vi "globalSetUp.vi"(8 "error in (no error)":errorcluster, 11 "Instrument Addon Host API Tests in":refnum<class "Instrument Addon Host API Tests.lvclass">) -> (0 "error out":errorcluster, 3 "Instrument Addon Host API Tests out":refnum<class "Instrument Addon Host API Tests.lvclass">)   [LabVIEW 2019, in "Instrument Addon Host API Tests.lvclass"]
uses:
  Instrument Addon Host API Tests.lvclass
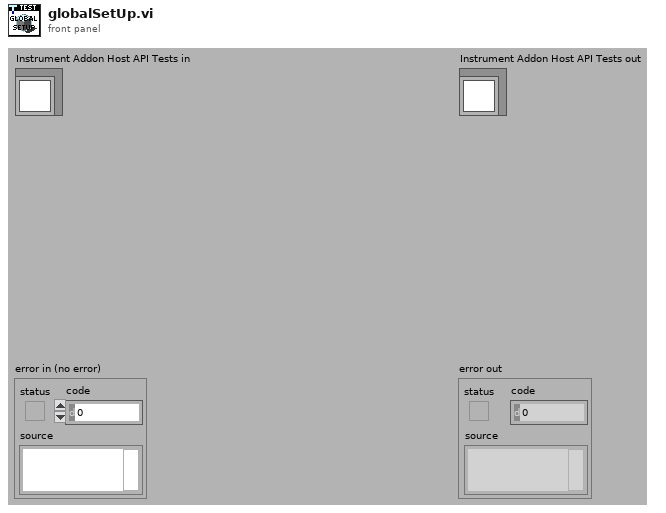
[diagram p1: front panel]
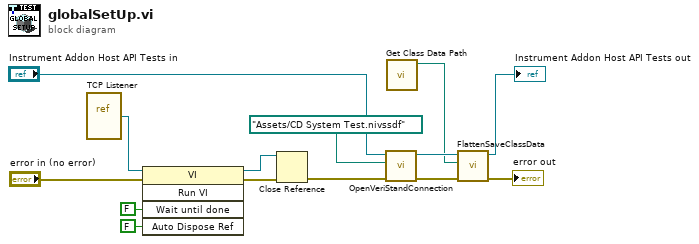
[diagram p0: block diagram]
diagram:
  n1 = vi-ref "TCP Listener.vi"() -> (w8:refnum<vi>)
  n2 = invoke class="VI" method="Run VI"(reference=w8, error in="error in (no error)", "Wait until done"=FALSE ("Wait Until Done"), "Auto Dispose Ref"=FALSE ("Auto Dispose Reference")) -> (reference out=w7:refnum<vi>, error out=w6:errorcluster)  [unwired: 1 in, 3 out]
  n3 = Close Reference(reference=w7, error in (no error)=w6) -> (error out=w2:errorcluster)
  n4 = call-dynamic "OpenVeriStandConnection.vi"("error in (no error)"=w2, "System Definition File"=path "Assets/CD System Test.nivssdf", "VeriStand Test Case in"="Instrument Addon Host API Tests in") -> ("error out"=w13:errorcluster, "VeriStand Test Case out"=w11:refnum<class "Instrument Addon Host API Tests.lvclass">)  [unwired: 6 in, 1 out]
  n5 = call "Get Class Data Path.vi"() -> ("Class Data File Path"=w1:path)  [unwired: 11 in]
  n6 = call-dynamic "FlattenSaveClassData.vi"("error in"=w13, "Class Data File Path"=w1, "VeriStandTestCase in"=w11) -> ("error out"=→"error out":errorcluster, "VeriStandTestCase out"=→"Instrument Addon Host API Tests out":refnum<class "Instrument Addon Host API Tests.lvclass">)  [unwired: 7 in]
